vi "NISE.Add Network Chassis.vi"(0 "SLSC Interface in":refnum<class "SLSC Interface.lvclass">, 1 "username":string, 2 "password":string, 5 "chassis IP address/hostname":string, 11 "error in (no error)":errorcluster, 12 "connect timeout (60 sec)":dbl=60.0) -> (4 "SLSC Interface out":refnum<class "SLSC Interface.lvclass">, 6 "chassis out":refnum<k21>, 15 "error out":errorcluster)   [LabVIEW 2016, in "SLSC Interface.lvclass"]
uses:
  SLSC Interface.lvclass
  SLSC Interface.lvclass/SLSC Interface.ctl
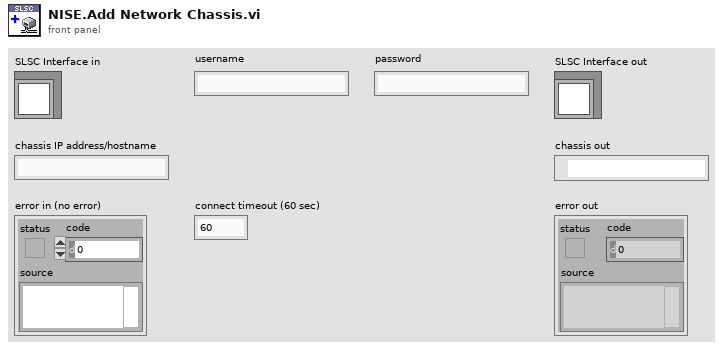
[diagram p1: front panel]
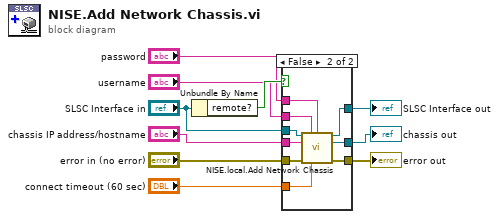
[diagram p0: block diagram]
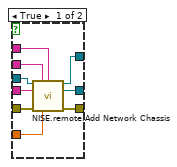
[diagram p2: hidden frame]
diagram:
  n1 = Unbundle By Name("SLSC Interface in") -> ("remote?"=w10:bool)
  n2 = case shown="False" w10 {
    tunnel: "SLSC Interface in" -> [w19 w28]
    tunnel: "username" -> [w18 w27]
    tunnel: "password" -> [w17 w26]
    tunnel: [w16 w25] -> w7
    tunnel: "chassis IP address/hostname" -> [w15 w24]
    tunnel: [w14 w23] -> w5
    tunnel: "error in (no error)" -> [w13 w22]
    tunnel: "connect timeout (60 sec)" -> [w12 w21]
    tunnel: [w11 w20] -> w2
    frame True {
      n3 = call "NISE.remote.Add Network Chassis.vi"("SLSC Remote in"=w19, "username"=w18, "password"=w17, "chassis IP address/hostname"=w15, "error in (no error)"=w13, "connect timeout (60 sec)"=w12) -> ("SLSC Remote out"=w16:refnum<class "SLSC Interface.lvclass">, "chassis out"=w14:refnum<k21>, "error out"=w11:errorcluster)  [unwired: 7 in]
    }
    frame False {
      n4 = call "NISE.local.Add Network Chassis.vi"("SLSC Local in"=w28, "username"=w27, "password"=w26, "chassis IP address/hostname"=w24, "error in (no error)"=w22, "connect timeout (60 sec)"=w21) -> ("SLSC Local out"=w25:refnum<class "SLSC Interface.lvclass">, "chassis out"=w23:refnum<k21>, "error out"=w20:errorcluster)  [unwired: 7 in]
    }
  }
  "error out" <- w2
  "SLSC Interface out" <- w7
  "chassis out" <- w5
